vi "midiInStart.vi"(8 "error in":errorcluster, 11 "midi in":refnum<class "midi.lvclass">) -> (0 "error out":errorcluster, 3 "midi out":refnum<class "midi.lvclass">)   [LabVIEW 2020, in "midi.lvclass"]
doc: "The midiInStart function starts MIDI input on the specified MIDI input device.\n\nThis function resets the time stamp to zero; time stamp values for subsequently received messages are relative to the time that this function was called. All messages except system-exclusive messages are sent directly to the client when they are received. System-exclusive messages are placed in the buffers supplied by the midiInAddBuffer function. If there are no buffers in the queue, the system-exclusive data is thrown away without notification to the client and input continues. Buffers are returned to the client when they are full, when a complete system-exclusive messagehas been received, or when the midiInReset function is used. The dwBytesRecorded member of the MIDIHDR structure will contain the actual length of data received. Calling this function when input is already started has no effect, and the function returns zero."
uses:
  midi.lvclass
  midi.lvclass/midi.ctl
  cpp-src/MIDIInToLabVIEWWrapper/x64/Release/MIDIInToLabVIEWWrapper.dll
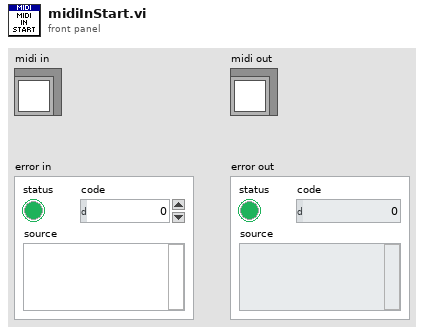
[diagram p1: front panel]
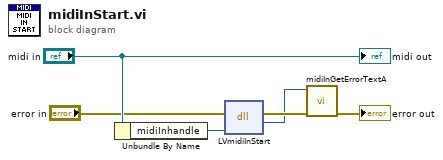
[diagram p0: block diagram]
diagram:
  n1 = Unbundle By Name("midi in") -> ("midiInhandle"=w1:u64)
  n2 = dll-call lib="C:/code/LabVIEW-MIDI/cpp-src/MIDIInToLabVIEWWrapper/x64/Release/MIDIInToLabVIEWWrapper.dll" fn="LVmidiInStart"(error in="error in", "hMidiIn"=w1) -> (error out=w4:errorcluster, "error"=w3:i32)  [unwired: 3 in, 1 out]
  n3 = call "midiInGetErrorTextA.vi"("error in"=w4, "Error Code"=w3) -> ("error out"=→"error out":errorcluster)  [unwired: 9 in]
  "midi out" <- "midi in"
